vi "2021 Advent puzzle 05.vi"() -> ()   [LabVIEW 2021]
panel:
  out "Count":i32
  out "Array":i16[][](array[numeric])
  out "min y":i32
  out "min x":i32
  out "max y":i32
  out "max x":i32
  out "Error in parsing input":errorcluster
  out "y2":i32[](array[numeric])
  out "x2":i32[](array[numeric])
  out "y1":i32[](array[numeric])
  out "x1":i32[](array[numeric])
  in  "Test":bool
  # "allow diag wron 21017 too low"
  # "Now I know the min and max values\nI can declare a 2D array 0..989 in both dimensions\nand fill it with numbers of a line hor or vert\nFor a horizontal row take the subset, add a one to each value \nand replace the subset\nfor each pair find out if it is hor or vert\nvertical is true when x1 is x2 Horizontal when y1=y2\nThe direction is a don't carre when the indexes need to swap."
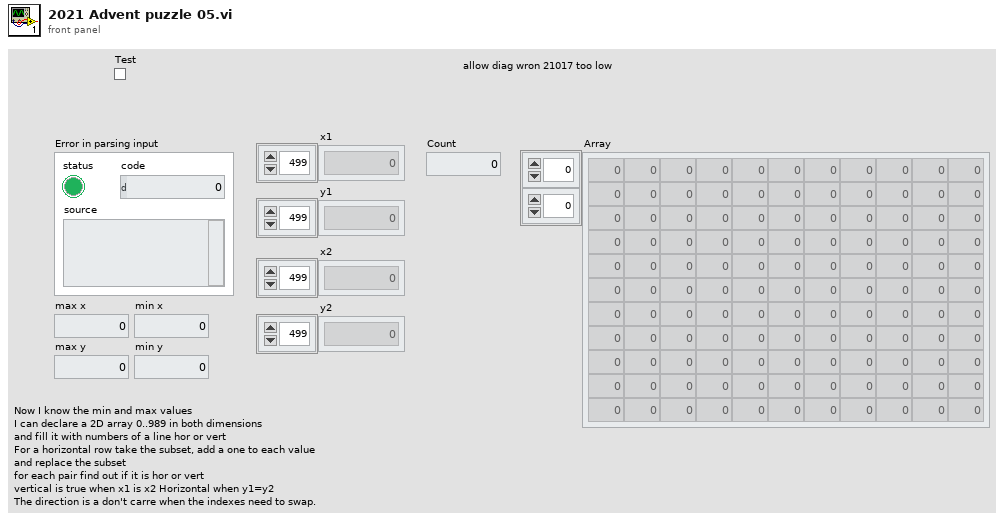
[diagram p1: front panel]
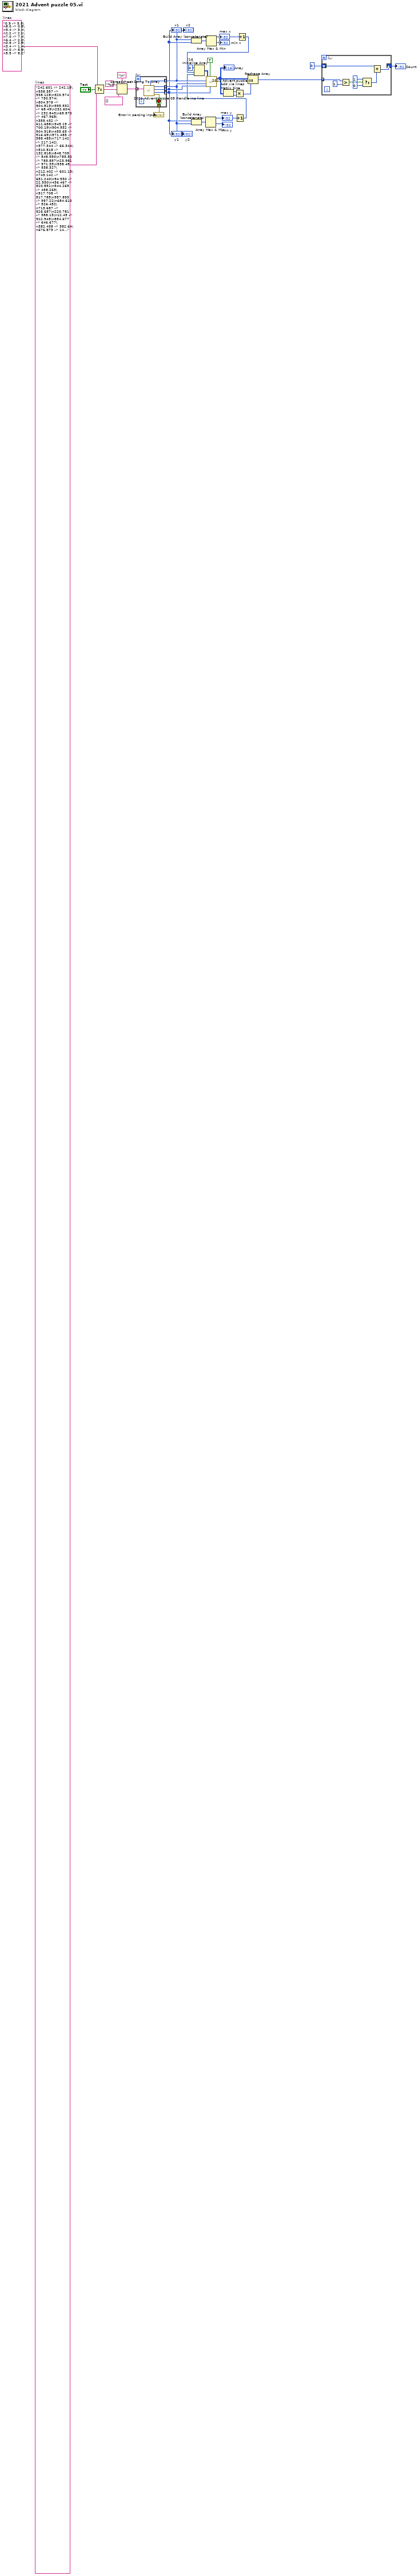
[diagram p0: block diagram]
diagram:
  w16 = i16 0  # I16
  w31 = "0,9 -> 5,9\n8,0 -> 0,8\n9,4 -> 3,4\n2,2 -> 2,1\n7,0 -> 7,4\n6,4 -> 2,0\n0,9 -> 2,9\n3,4 -> 1,4\n0,0 -> 8,8\n5,5 -> 8,2"  # lines
  w29 = "242,601 -> 242,18\n938,357 -> 938,128\n920,574 -> 750,574\n804,978 -> 804,813\n955,932 -> 68,45\n232,604 -> 232,843\n69,570 -> 467,968\n355,432 -> 611,688\n945,19 -> 700,19\n904,932 -> 904,918\n455,65 -> 516,65\n571,485 -> 588,485\n717,142 -> 217,142\n377,344 -> 66,344\n510,818 -> 132,818\n848,709 -> 848,950\n785,50 -> 785,857\n23,981 -> 971,33\n938,45 -> 938,327\n212,402 -> 601,13\n749,142 -> 651,240\n94,930 -> 22,930\n436,467 -> 820,851\n544,265 -> 458,265\n517,708 -> 517,785\n957,893 -> 957,22\n684,610 -> 526,452\n713,687 -> 526,687\n220,781 -> 988,13\n12,45 -> 912,945\n854,677 -> 646,677\n382,498 -> 382,64\n676,879 -> 148,351\n809,52 -> 336,525\n959,951 -> 41,33\n943,162 -> 132,973\n897,732 -> 897,308\n21,196 -> 702,877\n938,972 -> 656,972\n798,139 -> 90,847\n213,597 -> 582,966\n248,955 -> 973,230\n985,606 -> 985,885\n166,693 -> 804,693\n807,897 -> 28,118\n433,306 -> 433,447\n899,61 -> 60,900\n984,582 -> 691,582\n803,583 -> 910,583\n348,142 -> 348,244\n352,775 -> 352,430\n240,285 -> 240,406\n394,541 -> 394,655\n887,622 -> 298,33\n62,37 -> 861,836\n819,136 -> 29,926\n717,332 -> 717,408\n709,63 -> 276,496\n384,441 -> 150,441\n292,251 -> 557,516\n518,311 -> 52,777\n50,735 -> 479,306\n932,865 -> 139,72\n43,21 -> 982,960\n63,927 -> 796,194\n958,351 -> 958,623\n643,451 -> 35,451\n534,14 -> 459,14\n20,649 -> 924,649\n983,18 -> 35,966\n84,668 -> 203,668\n40,654 -> 748,654\n474,760 -> 85,371\n512,431 -> 272,431\n588,93 -> 112,569\n648,687 -> 832,687\n988,867 -> 116,867\n979,46 -> 94,931\n242,307 -> 800,865\n100,204 -> 807,911\n890,962 -> 88,962\n273,510 -> 273,201\n184,748 -> 813,119\n214,915 -> 950,179\n960,975 -> 89,104\n853,347 -> 853,79\n853,308 -> 884,308\n245,394 -> 245,640\n850,554 -> 604,800\n141,159 -> 141,378\n635,632 -> 897,894\n352,182 -> 550,182\n748,613 -> 748,887\n531,664 -> 255,388\n785,414 -> 432,767\n374,457 -> 653,736\n451,535 -> 444,535\n600,179 -> 434,13\n489,605 -> 845,961\n658,786 -> 658,196\n305,556 -> 305,914\n820,368 -> 204,984\n903,70 -> 548,425\n840,450 -> 796,494\n289,183 -> 768,662\n21,54 -> 950,983\n765,294 -> 209,850\n467,511 -> 703,747\n354,645 -> 730,645\n176,30 -> 964,818\n290,259 -> 345,259\n868,945 -> 96,173\n536,884 -> 536,94\n415,177 -> 415,99\n250,140 -> 466,140\n900,107 -> 900,249\n74,394 -> 137,394\n364,957 -> 364,81\n718,477 -> 718,227\n27,14 -> 988,975\n491,956 -> 154,956\n289,283 -> 289,225\n479,583 -> 604,583\n581,406 -> 23,964\n837,526 -> 732,526\n417,435 -> 417,206\n502,184 -> 20,666\n903,754 -> 817,668\n381,284 -> 967,870\n31,17 -> 176,17\n225,377 -> 179,377\n316,932 -> 358,890\n605,841 -> 559,841\n865,193 -> 865,827\n836,834 -> 142,140\n229,610 -> 232,610\n26,13 -> 872,859\n26,444 -> 26,79\n272,690 -> 531,949\n964,954 -> 331,954\n545,91 -> 335,91\n906,942 -> 906,301\n608,778 -> 608,364\n475,723 -> 475,710\n454,207 -> 614,207\n200,180 -> 917,897\n966,44 -> 71,939\n288,252 -> 288,413\n795,791 -> 66,62\n81,39 -> 588,546\n249,244 -> 892,244\n483,579 -> 853,579\n220,921 -> 220,286\n917,834 -> 675,834\n569,692 -> 569,521\n344,586 -> 835,95\n116,153 -> 888,925\n681,52 -> 871,242\n980,976 -> 27,23\n828,567 -> 482,567\n660,432 -> 660,441\n826,379 -> 280,379\n42,839 -> 259,622\n743,23 -> 91,23\n318,400 -> 318,528\n539,745 -> 734,940\n831,194 -> 831,210\n582,630 -> 361,851\n284,900 -> 213,829\n52,855 -> 763,855\n215,753 -> 452,753\n290,187 -> 417,187\n69,48 -> 69,126\n76,628 -> 76,365\n257,694 -> 54,694\n755,713 -> 556,912\n519,265 -> 342,265\n193,319 -> 193,651\n496,231 -> 900,231\n83,942 -> 83,524\n524,59 -> 989,524\n288,800 -> 907,181\n458,138 -> 586,138\n338,244 -> 934,840\n843,728 -> 843,476\n42,634 -> 657,19\n827,634 -> 369,176\n779,900 -> 779,503\n20,20 -> 870,870\n467,241 -> 467,142\n677,483 -> 501,483\n10,989 -> 989,10\n11,989 -> 989,11\n244,750 -> 244,607\n479,497 -> 48,928\n372,341 -> 615,341\n817,941 -> 339,941\n352,67 -> 352,581\n590,747 -> 590,405\n524,26 -> 524,37\n501,300 -> 117,300\n265,194 -> 491,420\n397,891 -> 983,305\n423,717 -> 423,922\n197,863 -> 197,217\n12,91 -> 379,91\n364,426 -> 364,185\n649,835 -> 649,309\n517,380 -> 485,380\n328,469 -> 568,469\n781,298 -> 781,264\n25,794 -> 25,197\n570,744 -> 570,544\n664,352 -> 632,320\n528,944 -> 528,696\n242,44 -> 900,702\n486,775 -> 486,556\n608,245 -> 788,245\n114,11 -> 114,508\n751,560 -> 751,884\n211,513 -> 448,513\n389,219 -> 308,300\n638,200 -> 105,200\n258,243 -> 365,243\n120,558 -> 556,122\n787,166 -> 274,166\n617,666 -> 185,234\n537,172 -> 808,172\n633,980 -> 282,980\n270,150 -> 270,225\n925,32 -> 48,909\n979,14 -> 891,102\n98,278 -> 98,485\n333,771 -> 119,771\n132,673 -> 132,189\n416,470 -> 482,404\n762,151 -> 925,151\n148,721 -> 378,491\n255,576 -> 255,474\n21,48 -> 938,965\n876,615 -> 777,615\n713,209 -> 209,209\n250,474 -> 271,453\n684,71 -> 451,71\n406,614 -> 519,501\n479,252 -> 112,252\n721,768 -> 284,331\n290,344 -> 290,111\n359,934 -> 544,934\n754,976 -> 726,976\n358,544 -> 358,904\n597,344 -> 597,581\n915,222 -> 915,255\n931,160 -> 135,956\n160,657 -> 348,657\n35,942 -> 949,28\n298,837 -> 298,356\n540,195 -> 540,119\n29,140 -> 29,955\n118,117 -> 980,979\n240,384 -> 464,608\n677,667 -> 361,351\n982,987 -> 11,16\n638,770 -> 95,227\n135,285 -> 135,349\n843,313 -> 843,529\n208,220 -> 945,957\n450,889 -> 977,362\n876,69 -> 283,69\n57,586 -> 57,231\n602,78 -> 602,564\n708,704 -> 267,704\n697,336 -> 697,264\n564,522 -> 519,567\n195,217 -> 274,138\n35,885 -> 116,804\n680,28 -> 148,28\n736,34 -> 736,616\n918,454 -> 52,454\n143,40 -> 415,40\n985,469 -> 985,282\n804,703 -> 107,703\n707,59 -> 296,470\n37,935 -> 931,41\n45,723 -> 45,531\n897,959 -> 165,227\n691,948 -> 523,948\n545,560 -> 545,45\n251,24 -> 748,521\n625,506 -> 625,626\n302,702 -> 989,15\n489,926 -> 489,507\n405,830 -> 405,871\n736,851 -> 19,134\n712,848 -> 48,184\n925,914 -> 33,22\n593,254 -> 369,478\n965,691 -> 155,691\n758,931 -> 349,522\n64,135 -> 820,891\n79,933 -> 79,683\n609,454 -> 233,454\n617,853 -> 309,545\n695,130 -> 695,578\n508,198 -> 363,198\n184,414 -> 275,505\n627,901 -> 519,901\n765,715 -> 213,715\n445,134 -> 669,134\n785,33 -> 302,516\n563,218 -> 470,125\n136,461 -> 264,461\n523,643 -> 674,643\n473,695 -> 473,235\n616,835 -> 757,976\n406,763 -> 406,224\n483,111 -> 203,111\n70,863 -> 922,11\n738,141 -> 738,54\n146,697 -> 332,883\n939,16 -> 23,932\n836,15 -> 317,534\n853,586 -> 853,596\n733,377 -> 733,461\n378,597 -> 378,640\n522,225 -> 522,78\n875,886 -> 875,130\n302,83 -> 771,83\n969,588 -> 419,38\n268,159 -> 585,476\n658,955 -> 33,330\n940,149 -> 492,149\n157,254 -> 962,254\n265,778 -> 265,365\n414,494 -> 608,494\n27,959 -> 948,38\n220,160 -> 220,891\n836,316 -> 836,179\n843,727 -> 163,47\n225,695 -> 598,695\n678,249 -> 892,249\n938,36 -> 938,170\n190,486 -> 40,336\n815,256 -> 815,866\n961,200 -> 961,89\n67,895 -> 67,853\n480,727 -> 852,727\n334,94 -> 334,452\n67,622 -> 987,622\n48,29 -> 982,963\n90,29 -> 963,902\n859,739 -> 338,739\n869,254 -> 474,649\n196,43 -> 69,43\n336,439 -> 336,837\n248,387 -> 587,48\n378,729 -> 162,513\n699,658 -> 513,844\n447,410 -> 670,410\n739,593 -> 889,443\n83,970 -> 964,89\n276,406 -> 276,191\n860,75 -> 247,688\n435,858 -> 435,905\n691,893 -> 691,757\n136,896 -> 611,421\n693,211 -> 477,427\n181,793 -> 181,717\n674,326 -> 664,336\n938,826 -> 164,52\n833,380 -> 833,753\n833,349 -> 230,952\n662,870 -> 662,23\n974,511 -> 145,511\n38,579 -> 57,579\n966,965 -> 966,498\n641,217 -> 240,618\n418,986 -> 834,986\n971,716 -> 971,263\n254,313 -> 254,823\n61,790 -> 61,834\n262,439 -> 262,864\n345,856 -> 894,307\n736,862 -> 281,862\n814,636 -> 814,240\n853,865 -> 853,22\n792,106 -> 207,106\n647,303 -> 531,303\n506,706 -> 337,706\n402,140 -> 402,958\n899,796 -> 669,796\n806,619 -> 463,276\n340,347 -> 340,363\n18,21 -> 979,982\n395,214 -> 395,862\n228,330 -> 333,330\n723,950 -> 723,150\n392,298 -> 36,298\n916,118 -> 114,920\n210,854 -> 80,724\n212,206 -> 513,507\n44,659 -> 161,659\n771,44 -> 198,617\n485,706 -> 169,706\n385,455 -> 308,455\n390,317 -> 390,385\n492,532 -> 56,968\n237,674 -> 712,674\n988,909 -> 254,175\n86,276 -> 448,276\n688,418 -> 927,179\n667,773 -> 504,610\n968,974 -> 109,115\n843,54 -> 843,265\n19,249 -> 19,437\n307,326 -> 341,360\n531,891 -> 531,202\n281,535 -> 270,546\n503,305 -> 164,644\n170,971 -> 30,971\n763,247 -> 946,247\n795,920 -> 623,920\n673,16 -> 899,16\n785,845 -> 290,845\n68,614 -> 68,711\n284,984 -> 67,984\n787,942 -> 120,942\n953,369 -> 773,549\n927,727 -> 315,115\n884,686 -> 254,56\n432,276 -> 432,287\n658,99 -> 81,676\n622,917 -> 679,917\n938,978 -> 938,793\n945,15 -> 369,15\n603,709 -> 603,74\n670,422 -> 222,870\n190,702 -> 190,362\n354,349 -> 369,334\n26,880 -> 876,30\n636,31 -> 636,731\n778,628 -> 778,25\n23,483 -> 170,483\n23,972 -> 963,32\n725,308 -> 384,308\n97,962 -> 620,962\n136,929 -> 136,768\n656,295 -> 851,295\n125,801 -> 755,171\n120,32 -> 553,32\n698,196 -> 286,608\n66,721 -> 66,836\n931,680 -> 931,499\n862,449 -> 862,743\n71,143 -> 180,252\n510,327 -> 612,225\n932,874 -> 352,874\n599,372 -> 583,372\n821,770 -> 126,75\n317,186 -> 495,186\n557,710 -> 56,209\n895,866 -> 306,277\n571,948 -> 571,738\n287,864 -> 243,864\n802,728 -> 802,198\n711,642 -> 983,642\n969,922 -> 969,645\n89,417 -> 57,385\n567,967 -> 567,781\n350,498 -> 142,498\n92,931 -> 988,35\n980,940 -> 152,112\n55,944 -> 679,320\n669,410 -> 669,679\n151,431 -> 241,431\n984,882 -> 80,882\n431,374 -> 431,39\n30,91 -> 765,826\n730,228 -> 80,878\n379,570 -> 705,570\n67,398 -> 67,136\n491,515 -> 491,344\n396,453 -> 749,453\n203,660 -> 203,579\n912,900 -> 912,280\n909,88 -> 367,88\n41,942 -> 825,158\n724,417 -> 17,417\n463,536 -> 170,536\n715,737 -> 715,134\n627,453 -> 805,453\n934,795 -> 695,556\n404,729 -> 738,729\n973,685 -> 973,310\n563,348 -> 771,556\n716,232 -> 983,232\n975,183 -> 975,759\n934,958 -> 117,958\n538,806 -> 538,84\n695,677 -> 629,677"  # lines
  n1 = Select(t=w31, s="Test", f=w29) -> (s? t:f=w25:string)
  n2 = Spreadsheet String To Array(delimiter (Tab)="\n", format string="%s", spreadsheet string=w25, array type (2D Dbl)=string[] []) -> (array=w24:string[])
  n3 = for {
    tunnel: w24 -> [w37] mode=indexing
    tunnel: [w36] -> w18 mode=indexing
    tunnel: [w35] -> w17 mode=indexing
    tunnel: [w34] -> w10 mode=indexing
    tunnel: [w33] -> w9 mode=indexing
    tunnel: [w32] -> w23
    stop <- w32 stop-if-true
    n4 = call "2021 Advent puzzle 05 Handle inp line.vi"("String"=w37) -> ("error out"=w32:errorcluster, "y2"=w33:i32, "x2"=w34:i32, "y1"=w35:i32, "x1"=w36:i32)  [unwired: 6 in]
  }
  "x1" <- w18
  "y1" <- w17
  "x2" <- w10
  "y2" <- w9
  "Error in parsing input" <- w23
  n5 = Build Array (concatenate)(w18, w10) -> (w22:i32[])
  n6 = Build Array (concatenate)(w9, w17) -> (w21:i32[])
  n7 = Array Max & Min(array=w21) -> (max value=w15:i32, min value=→"min y":i32)  [unwired: 2 out]
  "max y" <- w15
  n8 = Array Max & Min(array=w22) -> (max value=w14:i32, min value=→"min x":i32)  [unwired: 2 out]
  "max x" <- w14
  n9 = Increment(x=w15) -> (x+1=w11:i32)
  n10 = Increment(x=w14) -> (x+1=w12:i32)
  n11 = Initialize Array(w16, w12, w11) -> (w13:i16[][])
  n12 = call "2021 Advent puzzle 05 Add via lines.vi"("Y2"=w9, "Allow diag"=TRUE, "X2"=w10, "Y1"=w17, "X1"=w18, "Array in"=w13) -> ("Array out"=w8:i16[][])  [unwired: 5 in]
  "Array" <- w8
  n13 = Matrix Size(0:w8) -> (1:w7:i32, 2:w6:i32)
  n14 = Multiply(x=w7, y=w6) -> (x*y=w5:i32)
  n15 = Reshape Array(w8, w5) -> (w4:i16[])
  n16 = for {
    tunnel: w4 -> [w45] mode=indexing
    shift-right: [w38] -> w2
    shift-left: 0 -> [w40]
    n17 = Greater?(x=w45, y=i16 1) -> (0:w43:bool)
    n18 = Select(t=1, s=w43, f=0) -> (s? t:f=w39:i32)
    n19 = Add(x=w40, y=w39) -> (x+y=w38:i32)
  }
  "Count" <- w2
